vi "AboutMenu.vi"   [LabVIEW 2010]
panel:
  # "Java Internet LabVIEW Server 1.0\nEasy Java Simulations and LabVIEW connection \nCopyright (c) 2007 - UNED, Madrid - Spain\nCorresponding author: Héctor Vargas"
  # "Department of Computer Science and Automatic Control"
  # "In collaboration with Automatic Laboratory from EPFL, Switzerland"
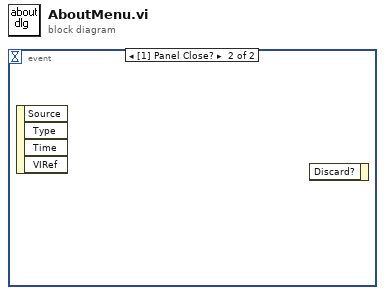
[diagram p0: block diagram]
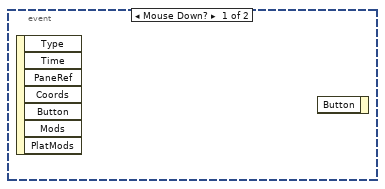
[diagram p2: hidden frame]
diagram:
  n1 = event shown="[1] Panel Close?" {
    selector: _ -> [_ _]
    dyn-events: _ -> [_ _]
    timeout: _ -> [_ _]
    event Mouse Down? {
      n2 = event-data() -> ()  [unwired: 8 out]
      n3 = event-data() -> ()  [unwired: 1 in, 2 out]
    }
    event Panel Close? {
      n4 = event-data() -> ()  [unwired: 5 out]
      n5 = event-data() -> ()  [unwired: 1 in, 2 out]
    }
  }
